vi "Experiment 2.VI"() -> ()   [LabVIEW 2017]
panel:
  out "Run Time (s)":dbl
  out "Iteration (ms)":u32
  in  "stop":bool
  out "Tank":dbl(slide) scale=0.0..10.0
  in  "Slide":dbl(slide) scale=0.0..10.0
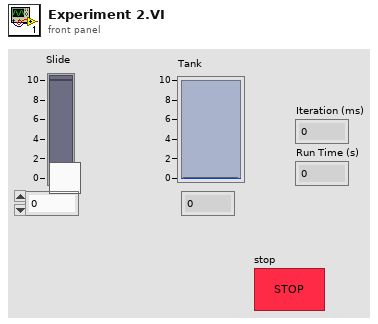
[diagram p1: front panel]
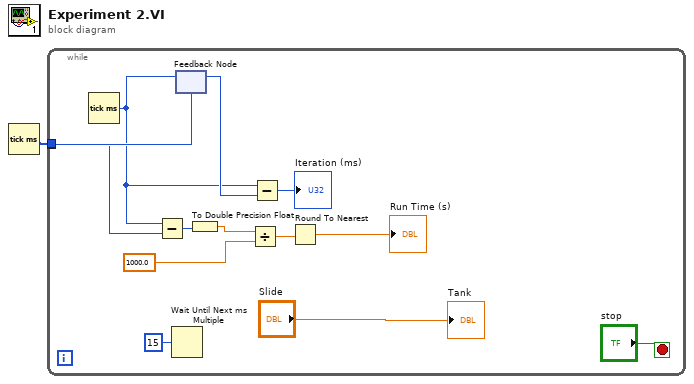
[diagram p0: block diagram]
diagram:
  n1 = Tick Count (ms)() -> (millisecond timer value=w1:u32)
  n2 = while {
    tunnel: w1 -> [w10]
    tunnel: w1 -> [w7]
    stop <- "stop" stop-if-true
    n3 = Tick Count (ms)() -> (millisecond timer value=w8:u32)
    n4 = Subtract(x=w8, y=w7) -> (x-y=w6:u32)
    n5 = Wait Until Next ms Multiple(millisecond multiple=u32 15) -> ()  [unwired: 1 out]
    n6 = feedback-in #1(w8) -> ()
    n7 = feedback #1(w10) -> (w11:u32)
    n8 = To Double Precision Float(number=w6) -> (double precision float=w5:dbl)
    n9 = Divide(x=w5, y=1000.0) -> (x/y=w3:dbl)
    n10 = Subtract(x=w8, y=w11) -> (x-y=→"Iteration (ms)":u32)
    n11 = Round To Nearest(number=w3) -> (nearest integer value=→"Run Time (s)":dbl)
    "Tank" <- "Slide"
  }
